vi "Test Window API.vi"(8 "error in (no error)":errorcluster) -> (0 "error out":errorcluster)   [LabVIEW 2015]
uses:
  <vilib>/addons/_JKI Toolkits/Caraya/classes/Test/Test.lvclass
  Window/Window.lvclass
  <vilib>/addons/_JKI Toolkits/Caraya/classes/Assert/Assert.lvclass
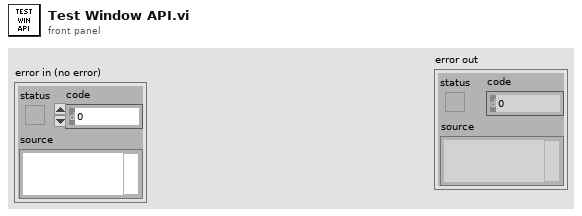
[diagram p1: front panel]
types:
  T1 = typedef "LVRectTypeDef.ctl" = cluster{"Left":i16, "Top":i16, "Right":i16, "Bottom":i16}
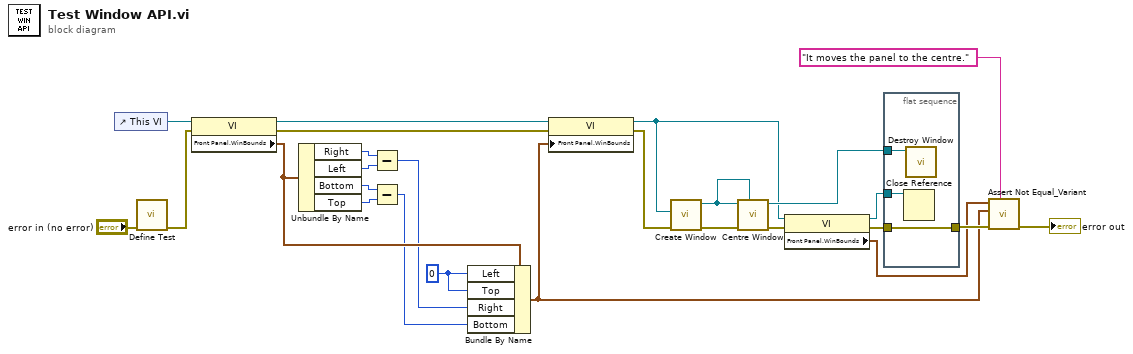
[diagram p0: block diagram]
diagram:
  w12 = i16 0 ("Left")
  n1 = control-ref of="This VI"() -> (w22:refnum<vi>)
  n2 = call <vilib>:"Define Test.vi"("error in (no error)"="error in (no error)") -> ("error out"=w16:errorcluster)  [unwired: 10 in]
  n3 = property class="VI"(reference=w22, error in=w16) -> (reference out=w21:refnum<vi>, error out=w15:errorcluster, "Front Panel.WinBounds"=w13:T1)
  n4 = Unbundle By Name(w13) -> ("Right"=w20:i16, "Left"=w19:i16, "Bottom"=w18:i16, "Top"=w17:i16)
  n5 = Subtract(x=w20, y=w19) -> (x-y=w11:i16)
  n6 = Subtract(x=w18, y=w17) -> (x-y=w10:i16)
  n7 = Bundle By Name(cluster=w13, "Left"=w12, "Top"=w12, "Right"=w11, "Bottom"=w10) -> (w3:T1)
  n8 = property class="VI"(reference=w21, error in=w15, "Front Panel.WinBounds"=w3) -> (reference out=w8:refnum<vi>, error out=w14:errorcluster)
  n9 = call "Create Window.vi"("error in (no error)"=w14, "Window"=w8) -> ("error out"=w25:errorcluster, "Window out"=w24:refnum<class "Window.lvclass">)  [unwired: 8 in]
  n10 = call "Centre Window.vi"("Parent Window"=w24, "error in (no error)"=w25, "Window in"=w24) -> ("error out"=w9:errorcluster, "Window out"=w23:refnum<class "Window.lvclass">)  [unwired: 7 in]
  n11 = property class="VI"(reference=w8, error in=w9) -> (reference out=w6:refnum<vi>, error out=w7:errorcluster, "Front Panel.WinBounds"=w2:T1)
  n12 = flat-sequence {
    tunnel: w23 -> [w29]
    tunnel: w7 -> [w27]
    tunnel: w6 -> [w28]
    tunnel: [w27] -> w5
    frame #0 {
      n13 = Close Reference(reference=w28) -> ()  [unwired: 1 in, 1 out]
      n14 = call "Destroy Window.vi"("Window in"=w29) -> ()  [unwired: 10 in, 1 out]
    }
  }
  n15 = call <vilib>:"Assert Not Equal_Variant.vi"("Label"="It moves the panel to the centre.", "error in (no error)"=w5, "Y"=w3, "X"=w2) -> ("error out"=→"error out":errorcluster)  [unwired: 7 in]
